vi "FGen Configuration.vi"(8 "error in (no error)":errorcluster) -> (0 "error out":errorcluster)   [LabVIEW 2021]
uses:
  Controls/FGen FGV Enum.ctl
  Controls/FGen Desktop Configuration.ctl
panel:
  in  "Cancel":bool
  in  "OK":bool
  in  "Step Interval (ms)":dbl
  in  "Step (Hz)":dbl
  in  "Stop Frequency (Hz)":dbl
  in  "Start Frequency (Hz)":dbl
  in  "Enable Sweep":bool
  in  "Offset (V)":dbl
  # "Sweep Settings"
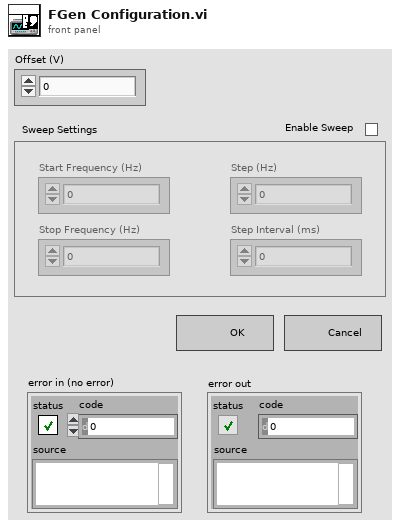
[diagram p1: front panel]
types:
  T1 = typedef "FGen FGV Enum.ctl" = enum16{"Set", "Get"}
  T2 = typedef "FGen Desktop Configuration.ctl" = cluster{"Offset (V)":dbl, "Enable Sweep":bool, "Start Frequency (Hz)":dbl, "Stop Frequency (Hz)":dbl, "Step (Hz)":dbl, "Step Interval (ms)":dbl, "Current Freq (Hz)":dbl, "Run":bool}
  T3 = enum8{"Enabled", "Disabled", "Disabled and Grayed Out"}
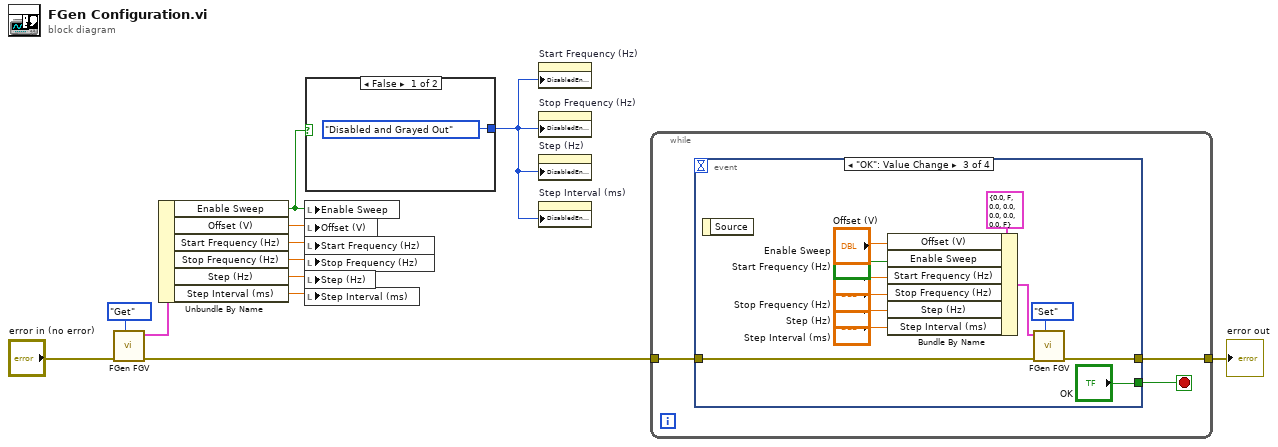
[diagram p0: block diagram]
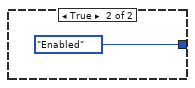
[diagram p2: hidden frame]
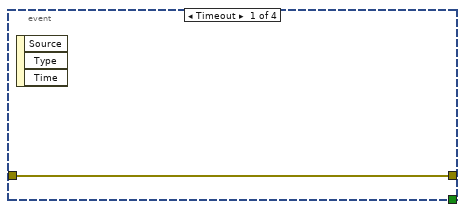
[diagram p3: hidden frame]
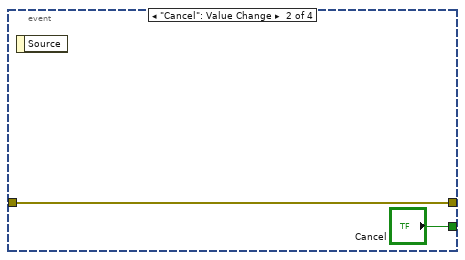
[diagram p4: hidden frame]
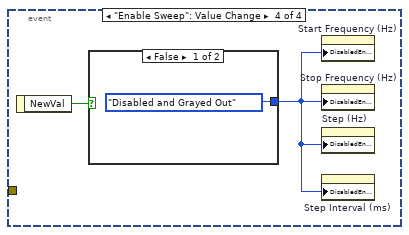
[diagram p5: hidden frame]
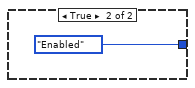
[diagram p6: hidden frame]
diagram:
  n1 = call "FGen FGV.vi"("Action"=FGen_FGV_Enum."Get", "error in (no error)"="error in (no error)") -> ("error out"=w12:errorcluster, "FGen Out"=w10:T2)  [unwired: 8 in]
  n2 = Unbundle By Name(w10) -> ("Enable Sweep"=w1:bool, "Offset (V)"=w9:dbl, "Start Frequency (Hz)"=w8:dbl, "Stop Frequency (Hz)"=w7:dbl, "Step (Hz)"=w6:dbl, "Step Interval (ms)"=w5:dbl)
  n3 = local write "Enable Sweep"(w1) -> ()
  n4 = local write "Offset (V)"(w9) -> ()
  n5 = local write "Start Frequency (Hz)"(w8) -> ()
  n6 = local write "Stop Frequency (Hz)"(w7) -> ()
  n7 = local write "Step (Hz)"(w6) -> ()
  n8 = local write "Step Interval (ms)"(w5) -> ()
  n9 = case shown="False" w1 {
    tunnel: [T3."Disabled and Grayed Out" ("Disabled") T3."Enabled" ("Disabled")] -> w2
    frame False {
    }
    frame True {
    }
  }
  n10 = property on="Start Frequency (Hz)" class="DigNum (strict)"("DisabledEnum"=w2) -> ()  [unwired: 2 in, 2 out]
  n11 = property on="Stop Frequency (Hz)" class="DigNum (strict)"("DisabledEnum"=w2) -> ()  [unwired: 2 in, 2 out]
  n12 = property on="Step (Hz)" class="DigNum (strict)"("DisabledEnum"=w2) -> ()  [unwired: 2 in, 2 out]
  n13 = property on="Step Interval (ms)" class="DigNum (strict)"("DisabledEnum"=w2) -> ()  [unwired: 2 in, 2 out]
  n14 = while {
    tunnel: w12 -> [w16]
    tunnel: [w15] -> w3
    stop <- w17 stop-if-true
    n15 = event shown="[2] \"OK\": Value Change" {
      selector: _ -> [_ _ _ _]
      dyn-events: _ -> [_ _ _ _]
      timeout: _ -> [_ _ _ _]
      tunnel: [_ "Cancel" "OK" _] -> w17
      tunnel: w16 -> [w18 w19 w23 _]
      tunnel: [w18 w19 w22 _] -> w15
      event Timeout {
        n16 = event-data() -> ()  [unwired: 1 in, 3 out]
      }
      event "Cancel": Value Change {
        n17 = event-data() -> ()  [unwired: 1 in, 1 out]
      }
      event "OK": Value Change {
        n18 = event-data() -> ()  [unwired: 1 in, 1 out]
        n19 = Bundle By Name(cluster=T2 {"Offset (V)"=0.0, "Enable Sweep"=FALSE, "Start Frequency (Hz)"=0.0, "Stop Frequency (Hz)"=0.0, "Step (Hz)"=0.0, "Step Interval (ms)"=0.0, "Current Freq (Hz)"=0.0, "Run"=FALSE} ("FGen"), "Offset (V)"="Offset (V)", "Enable Sweep"="Enable Sweep", "Start Frequency (Hz)"="Start Frequency (Hz)", "Stop Frequency (Hz)"="Stop Frequency (Hz)", "Step (Hz)"="Step (Hz)", "Step Interval (ms)"="Step Interval (ms)") -> (w24:T2)
        n20 = call "FGen FGV.vi"("Action"=FGen_FGV_Enum."Set", "error in (no error)"=w23, "FGen"=w24) -> ("error out"=w22:errorcluster)  [unwired: 7 in, 1 out]
      }
      event "Enable Sweep": Value Change {
        n21 = event-data() -> ("NewVal"=w34:bool)  [unwired: 1 in]
        n22 = case shown="False" w34 {
          tunnel: [T3."Disabled and Grayed Out" ("Disabled") T3."Enabled" ("Disabled")] -> w33
          frame False {
          }
          frame True {
          }
        }
        n23 = property on="Start Frequency (Hz)" class="DigNum (strict)"("DisabledEnum"=w33) -> ()  [unwired: 2 in, 2 out]
        n24 = property on="Stop Frequency (Hz)" class="DigNum (strict)"("DisabledEnum"=w33) -> ()  [unwired: 2 in, 2 out]
        n25 = property on="Step (Hz)" class="DigNum (strict)"("DisabledEnum"=w33) -> ()  [unwired: 2 in, 2 out]
        n26 = property on="Step Interval (ms)" class="DigNum (strict)"("DisabledEnum"=w33) -> ()  [unwired: 2 in, 2 out]
      }
    }
  }
  "error out" <- w3
